vi "Picture Point to XY.vi"(10 "scaling info":T1={"pixels per unit"=1.0, "fit radius (units)"=1.0, "center point (pixels)"={"x"=0, "y"=0}}, 11 "xy point (pixels)":cluster{"x":i16, "y":i16}) -> (3 "xy point (units)":cluster{"x":dbl, "y":dbl})   [LabVIEW 2017, in "NI_Robotics_2D Rangefinder Picture.lvlib"]
uses:
  <vilib>/robotics/Controls/2D Rangefinder/2D Rangefinder Picture/NI_Robotics_2D Rangefinder Picture.lvlib
  <vilib>/robotics/Controls/2D Rangefinder/2D Rangefinder Picture/Scaling Info.ctl
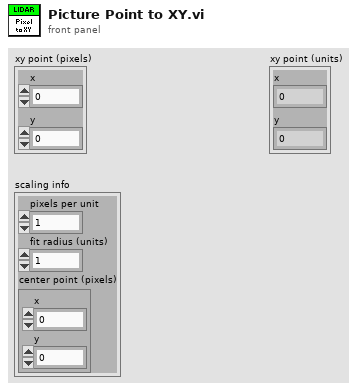
[diagram p1: front panel]
types:
  T1 = typedef "NI_Robotics_2D Rangefinder Picture.lvlib/Scaling Info.ctl" = cluster{"pixels per unit":dbl, "fit radius (units)":dbl, "center point (pixels)":cluster{"x":i16, "y":i16}}
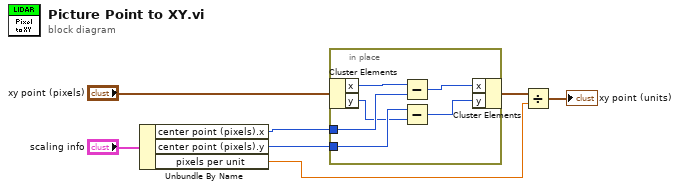
[diagram p0: block diagram]
diagram:
  n1 = Unbundle By Name("scaling info") -> ("center point (pixels).x"=w6:i16, "center point (pixels).y"=w5:i16, "pixels per unit"=w2:dbl)
  n2 = in-place {
    in-place-border: w6 -> [w12]
    in-place-border: w5 -> [w10]
    n3 = in-place-cluster #1("xy point (pixels)") -> ("x"=w13:i16, "y"=w9:i16)
    n4 = Subtract(x=w13, y=w12) -> (x-y=w11:i16)
    n5 = Subtract(x=w10, y=w9) -> (x-y=w8:i16)
    n6 = in-place-cluster #1("x"=w11, "y"=w8) -> (w3:cluster{"x":i16, "y":i16})
  }
  n7 = Divide(x=w3, y=w2) -> (x/y=→"xy point (units)":cluster{"x":dbl, "y":dbl})
